vi "smu_setup.vi"(8 "error in (no error)":errorcluster, 10 "Measurement settings":T1 {"Voltage range" items=["Auto", "200 mV", "2.1 V", "21 V", "210 V"]; "Enable display" items=["False", "True"]; "Auto settling delay" items=["False", "True"]; "Settling delay (ms)" min=0.2 max=999999.9; "Integration time (NPLC)" items=["0.01", "0.1", "1", "10"]; "Current range" items=["Auto", "1 uA", "10 uA", "100 uA", "1 mA", "10 mA", "100 mA", "1 A"]; "Dual JV sweep" items=["False", "True"]; "JV sweep direction" items=["Ascending", "Descending"]; "JV voltage step (V)" min=0.0001 max=5.0 step=0.0001; "Solar cell measurement mode" items=["J-V", "Voc", "Jsc"]; "LED current sweep direction" items=["Ascending", "Descending"]; "LED current sweep mode" items=["Linear", "Logarithmic"]; "Maximum LED Current (A)" min=0.0 max=0.7 step=0.001 format="%#.3f"; "Minimum LED current (A)" min=0.0 max=0.7 step=0.001 format="%#.3f"}, 11 "VISA Refnum in":refnum<visa-resource-name>) -> (0 "error out":errorcluster, 1 "Measure Mode":u16, 2 "Source Mode":u16, 3 "VISA resource name out":refnum<visa-resource-name>, 4 "Range":dbl, 5 "samples":i32)   [LabVIEW 2018]
uses:
  typedefs/measurement_settings.ctl
  <vilib>/Analysis/1siggen.llb/Ramp Pattern by Delta.vi
  <instrlib>/Keithley 24XX/Keithley 24XX.lvlib
  <vilib>/Analysis/NI_AALBase.lvlib
panel:
  out "Autorange":bool
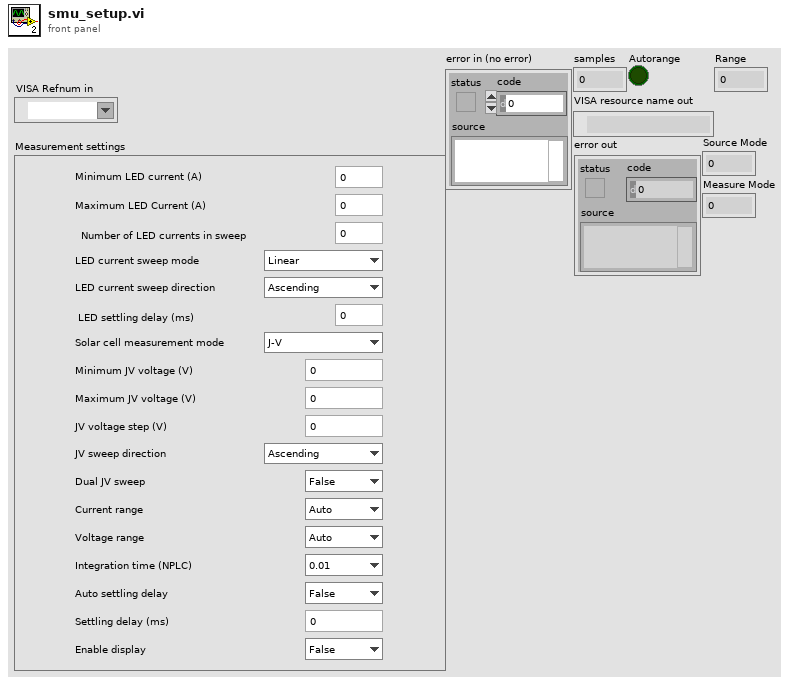
[diagram p1: front panel]
types:
  T1 = typedef "measurement_settings.ctl" = cluster{"Minimum LED current (A)":dbl, "Maximum LED Current (A)":dbl, "Number of LED currents in sweep":u32, "LED current sweep mode":u16, "LED current sweep direction":u16, "LED settling delay (ms)":u32, "Solar cell measurement mode":u16, "Minimum JV voltage (V)":dbl, "Maximum JV voltage (V)":dbl, "JV voltage step (V)":dbl, "JV sweep direction":u16, "Dual JV sweep":u16, "Current range":u16, "Voltage range":u16, "Integration time (NPLC)":u16, "Auto settling delay":u16, "Settling delay (ms)":dbl, "Enable display":u16}
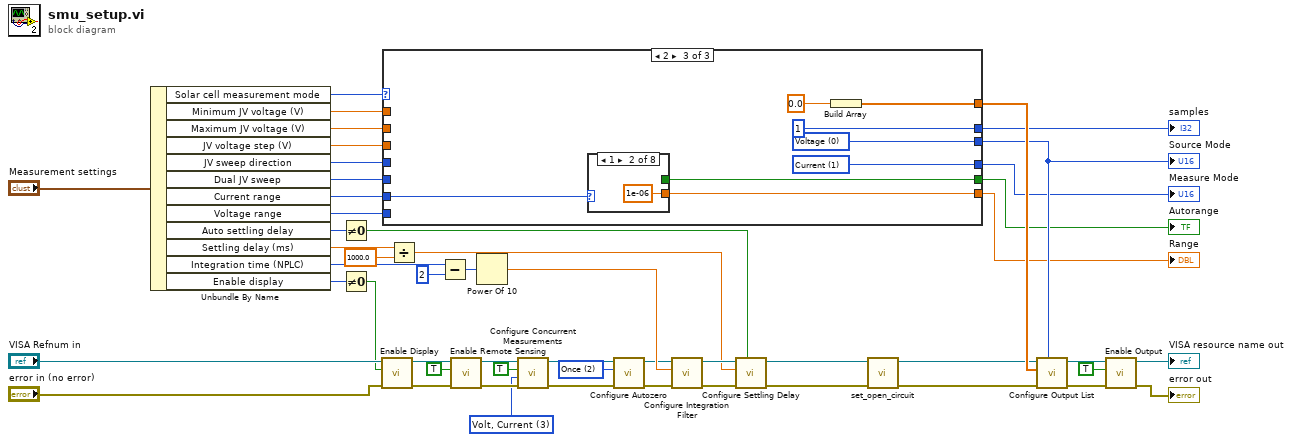
[diagram p0: block diagram]
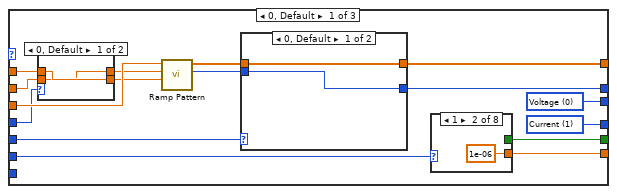
[diagram p2: hidden frame]
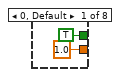
[diagram p3: hidden frame]
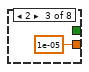
[diagram p4: hidden frame]
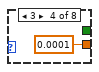
[diagram p5: hidden frame]
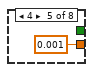
[diagram p6: hidden frame]
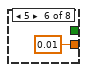
[diagram p7: hidden frame]
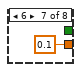
[diagram p8: hidden frame]
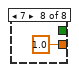
[diagram p9: hidden frame]
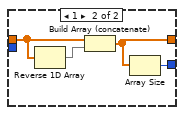
[diagram p10: hidden frame]
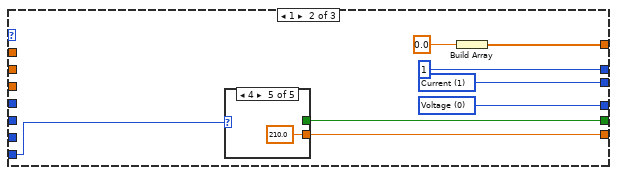
[diagram p12: hidden frame]
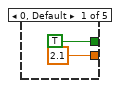
[diagram p13: hidden frame]
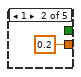
[diagram p14: hidden frame]
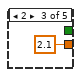
[diagram p15: hidden frame]
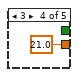
[diagram p16: hidden frame]
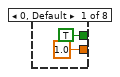
[diagram p17: hidden frame]
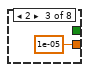
[diagram p18: hidden frame]
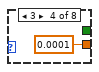
[diagram p19: hidden frame]
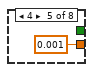
[diagram p20: hidden frame]
diagram:
  w33 = u16 2 items=["On", "Off", "Once"] ("Autozero  (0: On)")
  w34 = u16 3 items=["Volts", "Current", "Resistance", "Volt, Current", "Volts, Resistance", "Current, Resistance", "All"] ("Measurement Selection (3: Volts, Current)")
  n1 = Unbundle By Name("Measurement settings") -> ("Solar cell measurement mode"=w20:u16, "Minimum JV voltage (V)"=w17:dbl, "Maximum JV voltage (V)"=w16:dbl, "JV voltage step (V)"=w19:dbl, "JV sweep direction"=w18:u16, "Dual JV sweep"=w15:u16, "Current range"=w12:u16, "Voltage range"=w11:u16, "Auto settling delay"=w27:u16, "Settling delay (ms)"=w25:dbl, "Integration time (NPLC)"=w32:u16, "Enable display"=w38:u16)
  n2 = Not Equal To 0?(x=w27) -> (x != 0?=w26:bool)
  n3 = Not Equal To 0?(x=w38) -> (x != 0?=w37:bool)
  n4 = call <instrlib>:"Enable Display.vi"("error in (no error)"="error in (no error)", "Enable Display (T: Enable)"=w37, "VISA resource name"="VISA Refnum in") -> ("error out"=w46:errorcluster, "VISA resource name out"=w43:refnum<visa-resource-name>)  [unwired: 7 out]
  n5 = case shown="2" w20 {
    tunnel: w19 -> [w67 _ _]
    tunnel: w18 -> [w66 _ _]
    tunnel: w17 -> [w65 _ _]
    tunnel: w16 -> [w64 _ _]
    tunnel: w15 -> [w60 _ _]
    tunnel: [w58 w91 w105] -> w14
    tunnel: [w57 1 ("samples") 1 ("samples")] -> w13
    tunnel: [w56 w94 w108] -> w10
    tunnel: w12 -> [w55 _ w101]
    tunnel: w11 -> [_ w89 _]
    tunnel: [w54 w90 w104] -> w9
    tunnel: [w53 w87 w102] -> w2
    tunnel: [w52 w88 w103] -> w1
    frame 0, Default {
      w54 = u16 1 items=["Voltage", "Current"] ("Source Mode  (0: Voltage)")
      w56 = u16 0 items=["Voltage", "Current"] ("Source Mode  (0: Voltage)")
      n6 = case shown="0, Default" w66 {
        tunnel: w65 -> [w84 w86]
        tunnel: w64 -> [w83 w85]
        tunnel: [w83 w86] -> w63
        tunnel: [w84 w85] -> w62
        frame 0, Default {
        }
        frame 1 {
        }
      }
      n7 = call-poly <vilib>:"Ramp Pattern.vi"("start"=w62, "end"=w63, "delta"=w67) -> ("samples"=w59:i32, "Ramp Pattern"=w61:dbl[])  [unwired: 6 in, 1 out]
      n8 = case shown="0, Default" w60 {
        tunnel: w61 -> [w78 w81]
        tunnel: [w78 w80] -> w58
        tunnel: [w77 w79] -> w57
        tunnel: w59 -> [w77 _]
        frame 0, Default {
        }
        frame 1 {
          n9 = Reverse 1D Array(array=w81) -> (reversed array=w82:dbl[])
          n10 = Build Array (concatenate)(w81, w82) -> (w80:dbl[])
          n11 = Array Size(array=w80) -> (size(s)=w79:i32)
        }
      }
      n12 = case shown="1" w55 {
        tunnel: [1.0 ("Output Level (0)") 1e-06 ("Output Level (0)") 1e-05 ("Output Level (0)") 0.0001 ("Output Level (0)") 0.001 ("Output Level (0)") 0.01 ("Output Level (0)") 0.1 ("Output Level (0)") 1.0 ("Output Level (0)")] -> w53
        tunnel: [TRUE _ _ _ _ _ _ _] -> w52
        frame 0, Default {
        }
        frame 1 {
        }
        frame 2 {
        }
        frame 3 {
        }
        frame 4 {
        }
        frame 5 {
        }
        frame 6 {
        }
        frame 7 {
        }
      }
    }
    frame 1 {
      w90 = u16 0 items=["Voltage", "Current"] ("Source Mode  (0: Voltage)")
      w94 = u16 1 items=["Voltage", "Current"] ("Source Mode  (0: Voltage)")
      n13 = case shown="4" w89 {
        tunnel: [TRUE _ _ _ _] -> w88
        tunnel: [2.1 ("Output Level (0)") 0.2 ("Output Level (0)") 2.1 ("Output Level (0)") 21.0 ("Output Level (0)") 210.0 ("Output Level (0)")] -> w87
        frame 0, Default {
        }
        frame 1 {
        }
        frame 2 {
        }
        frame 3 {
        }
        frame 4 {
        }
      }
      n14 = Build Array(0.0 ("element")) -> (w91:dbl[])
    }
    frame 2 {
      w104 = u16 1 items=["Voltage", "Current"] ("Source Mode  (0: Voltage)")
      w108 = u16 0 items=["Voltage", "Current"] ("Source Mode  (0: Voltage)")
      n15 = case shown="1" w101 {
        tunnel: [1.0 ("Output Level (0)") 1e-06 ("Output Level (0)") 1e-05 ("Output Level (0)") 0.0001 ("Output Level (0)") 0.001 ("Output Level (0)") 0.01 ("Output Level (0)") 0.1 ("Output Level (0)") 1.0 ("Output Level (0)")] -> w102
        tunnel: [TRUE _ _ _ _ _ _ _] -> w103
        frame 0, Default {
        }
        frame 1 {
        }
        frame 2 {
        }
        frame 3 {
        }
        frame 4 {
        }
        frame 5 {
        }
        frame 6 {
        }
        frame 7 {
        }
      }
      n16 = Build Array(0.0 ("element")) -> (w105:dbl[])
    }
  }
  "samples" <- w13
  "Range" <- w2
  "Autorange" <- w1
  "Source Mode" <- w10
  "Measure Mode" <- w9
  n17 = Divide(x=w25, y=1000.0 ("x")) -> (x/y=w23:dbl)
  n18 = Subtract(x=w32, y=u16 2) -> (x-y=w30:u16)
  n19 = call <instrlib>:"Enable Remote Sensing.vi"("error in (no error)"=w46, "Enable Remote Sensing (T: Enable)"=TRUE, "VISA resource name"=w43) -> ("error out"=w45:errorcluster, "VISA resource name out"=w44:refnum<visa-resource-name>)  [unwired: 7 in]
  n20 = Power Of 10(x=w30) -> (10^x=w29:dbl)
  n21 = call <instrlib>:"Configure Concurrent Measurements.vi"("error in (no error)"=w45, "Measurement Selection (3: Volts, Current)"=w34, "Enable Concurrent Measurements (F: Disable)"=TRUE, "VISA resource name"=w44) -> ("error out"=w42:errorcluster, "VISA resource name out"=w41:refnum<visa-resource-name>)  [unwired: 6 in]
  n22 = call <instrlib>:"Configure Autozero.vi"("error in (no error)"=w42, "Autozero  (0: On)"=w33, "VISA resource name"=w41) -> ("error out"=w51:errorcluster, "VISA resource name out"=w28:refnum<visa-resource-name>)  [unwired: 7 in]
  n23 = call <instrlib>:"Configure Integration Filter.vi"("error in (no error)"=w51, "Measurement Speed (1 PLC)"=w29, "VISA resource name"=w28) -> ("error out"=w50:errorcluster, "VISA resource name out"=w49:refnum<visa-resource-name>)  [unwired: 7 in]
  n24 = call <instrlib>:"Configure Settling Delay.vi"("Auto Settle (T: Enable)"=w26, "error in (no error)"=w50, "Manual Settling Delay (0 sec)"=w23, "VISA resource name"=w49) -> ("error out"=w21:errorcluster, "VISA resource name out"=w22:refnum<visa-resource-name>)  [unwired: 6 in]
  n25 = call "set_open_circuit.vi"("error in (no error)"=w21, "VISA Refnum in"=w22) -> ("error out"=w7:errorcluster, "VISA Refnum out"=w8:refnum<visa-resource-name>)  [unwired: 8 in]
  n26 = call <instrlib>:"Configure Output List.vi"("Source Mode  (0: Voltage)"=w10, "error in (no error)"=w7, "Output List"=w14, "VISA resource name"=w8) -> ("error out"=w5:errorcluster, "VISA resource name out"=w6:refnum<visa-resource-name>)  [unwired: 6 in]
  n27 = call <instrlib>:"Enable Output.vi"("error in (no error)"=w5, "Enable Output (T: Enable)"=TRUE, "VISA resource name"=w6) -> ("error out"=→"error out":errorcluster, "VISA resource name out"=→"VISA resource name out":refnum<visa-resource-name>)  [unwired: 7 in]
